vi "dequeue_command.vi"(8 "error in (no error)":errorcluster caption="错误输入（无错误）", 11 "OneMotion输入":refnum<class "OneMotion.lvclass">) -> (0 "error out":errorcluster caption="错误输出", 2 "command":cluster{"cmd":T1, "cmd data":variant}, 3 "OneMotion输出":refnum<class "OneMotion.lvclass">)   [LabVIEW 2016, in "MotionControl.lvlib" / "OneMotion.lvclass"]
uses:
  <userlib>/MotionControl/OneMotion/OneMotion.lvclass
  <userlib>/MotionControl/OneMotion/cmd_motion.ctl
  <userlib>/MotionControl/OneMotion/OneMotion.lvclass/OneMotion.ctl
  <userlib>/MotionControl/MotionControl.lvlib
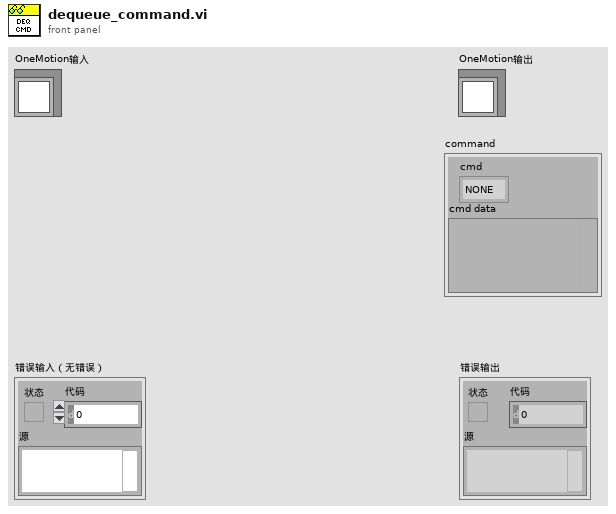
[diagram p1: front panel]
types:
  T1 = typedef "MotionControl.lvlib/OneMotion.lvclass/cmd_motion.ctl" = enum16{"NONE", "MOVE_MOTION", "EXIT", "STP_MOTION", "SPEED_MOTION", "WAIT_FOR_S3", "WAIT_A_TIME", "SKIP"}
  T2 = typedef "MotionControl.lvlib/OneMotion.lvclass/unit mode.ctl" = enum16{"motor (pulse)", "linear (mm) or radial (degree)"}
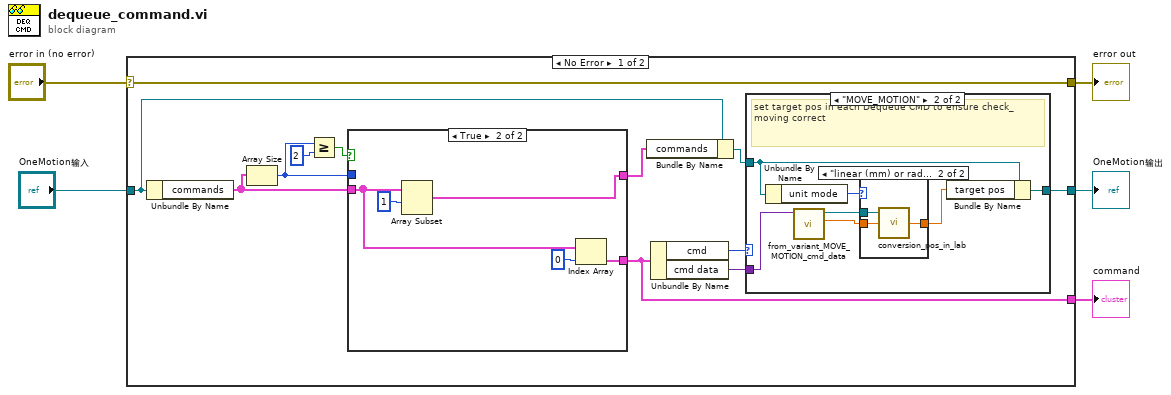
[diagram p0: block diagram]
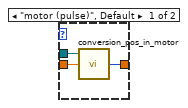
[diagram p3: hidden frame]
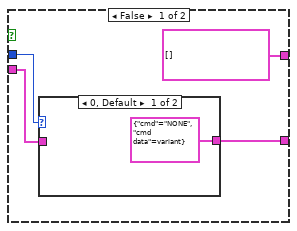
[diagram p4: hidden frame]
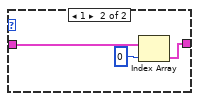
[diagram p5: hidden frame]
diagram:
  n1 = case shown="No Error" "error in (no error)" {
    selector: "error in (no error)" -> [w17 w45]
    tunnel: [w17 w45] -> w4
    tunnel: [w6 w46] -> w2
    tunnel: "OneMotion输入" -> [w12 w46]
    tunnel: [w10 _] -> w1
    frame No Error {
      n2 = Unbundle By Name(w12) -> ("commands"=w16:cluster{"cmd":T1, "cmd data":variant}[])
      n3 = Array Size(array=w16) -> (size(s)=w13:i32)
      n4 = Greater Or Equal?(x=w13, y=2) -> (x >= y?=w14:bool)
      n5 = case shown="True" w14 {
        tunnel: [w34 w43] -> w10
        tunnel: w16 -> [w33 w42]
        tunnel: w13 -> [w35 _]
        tunnel: [cluster{"cmd":T1, "cmd data":variant}[] [] w40] -> w11
        frame False {
          n6 = case shown="0, Default" w35 {
            tunnel: [cluster{"cmd":T1, "cmd data":variant} {"cmd"=enum."NONE", "cmd data"=variant} ("command") w37] -> w34
            tunnel: w33 -> [_ w38]
            frame 0, Default {
            }
            frame 1 {
              n7 = Index Array(array=w38, index=0 ("索引")) -> (element=w37:cluster{"cmd":T1, "cmd data":variant})
            }
          }
        }
        frame True {
          n8 = Array Subset(array=w42, index=1 ("索引")) -> (w40:cluster{"cmd":T1, "cmd data":variant}[])  [unwired: 1 in]
          n9 = Index Array(array=w42, index=0 ("索引")) -> (element=w43:cluster{"cmd":T1, "cmd data":variant})
        }
      }
      n10 = Bundle By Name(cluster=w12, "commands"=w11) -> (w7:refnum<class "OneMotion.lvclass">)
      n11 = Unbundle By Name(w10) -> ("cmd"=w9:T1, "cmd data"=w8:variant)
      n12 = case shown="\"MOVE_MOTION\"" w9 {
        tunnel: w8 -> [_ w25]
        tunnel: w7 -> [w18 w21]
        tunnel: [w18 w19] -> w6
        frame "NONE", Default {
        }
        frame "MOVE_MOTION" {
          # "set target pos in each Dequeue CMD to ensure check_moving correct"
          n13 = Unbundle By Name(w21) -> ("unit mode"=w24:T2)
          n14 = call <userlib>:"from_variant_MOVE_MOTION_cmd_data.vi"("variant"=w25) -> ("target pos"=w22:dbl, "OneMotion.lvclass"=w23:refnum<class "OneMotion.lvclass">)  [unwired: 9 in]
          n15 = case shown="\"linear (mm) or radial (degree)\"" w24 {
            tunnel: w23 -> [w28 w31]
            tunnel: w22 -> [w27 w30]
            tunnel: [w26 w29] -> w20
            frame "motor (pulse)", Default {
              n16 = call <userlib>:"conversion_pos_in_motor.vi"("pos"=w27, "OneMotion 输入"=w28) -> ("pos in motor"=w26:i32)  [unwired: 1 in, 2 out]
            }
            frame "linear (mm) or radial (degree)" {
              n17 = call <userlib>:"conversion_pos_in_lab.vi"("pos"=w30, "OneMotion 输入"=w31) -> ("pos in lab"=w29:dbl)  [unwired: 1 in, 2 out]
            }
          }
          n18 = Bundle By Name(cluster=w21, "target pos"=w20) -> (w19:refnum<class "OneMotion.lvclass">)
        }
      }
    }
    frame Error {
    }
  }
  "error out" <- w4
  "OneMotion输出" <- w2
  "command" <- w1
